vi "Read String Assertion Type.vi"(8 "error in (no error)":errorcluster, 11 "String Assertion in":refnum<class "String Assertion.lvclass">) -> (0 "error out":errorcluster, 2 "String Assertion Type":T1, 3 "String Assertion out":refnum<class "String Assertion.lvclass">)   [LabVIEW 2020, in "MacroAssert.lvlib" / "String Assertion.lvclass"]
uses:
  String Assertion.lvclass
  String Assertion.lvclass/String Assertion.ctl
  String Assertion Type.ctl
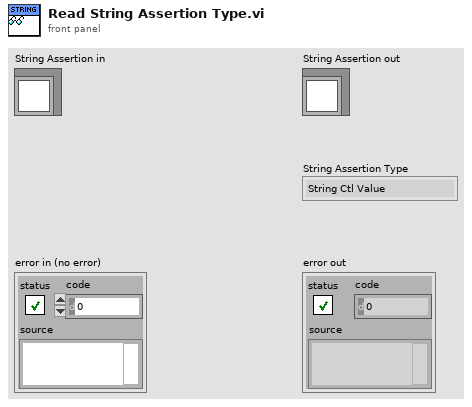
[diagram p1: front panel]
types:
  T1 = typedef "MacroAssert.lvlib/String Assertion.lvclass/String Assertion Type.ctl" = enum16{"String Ctl Value", "Ctl Caption Property", "Ctl Tip Strip Property", "Frontmost VI Name", "Frontmost Window Name"}
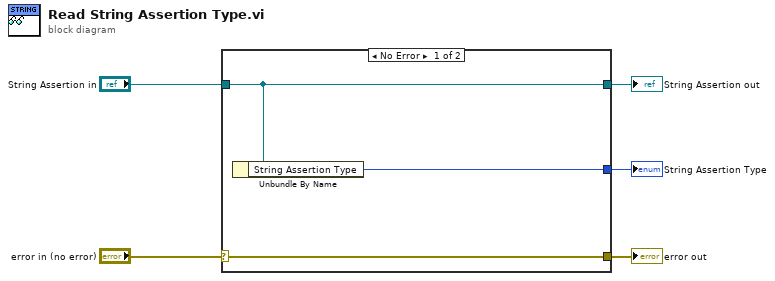
[diagram p0: block diagram]
diagram:
  n1 = case shown="No Error" "error in (no error)" {
    selector: "error in (no error)" -> [w8 w9]
    tunnel: [w8 w9] -> w4
    tunnel: [w7 w10] -> w2
    tunnel: "String Assertion in" -> [w7 w10]
    tunnel: [w6 _] -> w1
    frame No Error {
      n2 = Unbundle By Name(w7) -> ("String Assertion Type"=w6:T1)
    }
    frame Error {
    }
  }
  "error out" <- w4
  "String Assertion out" <- w2
  "String Assertion Type" <- w1
